vi "模式插入面板.vi"(10 "面板地址":string(combo), 11 "模式选择":string(combo)) -> ()   [LabVIEW 2019]
panel:
  in  "模式input":T1 {"pannel"."ID" format="%02x"}
  in  "节点列表":T2(array[cluster])
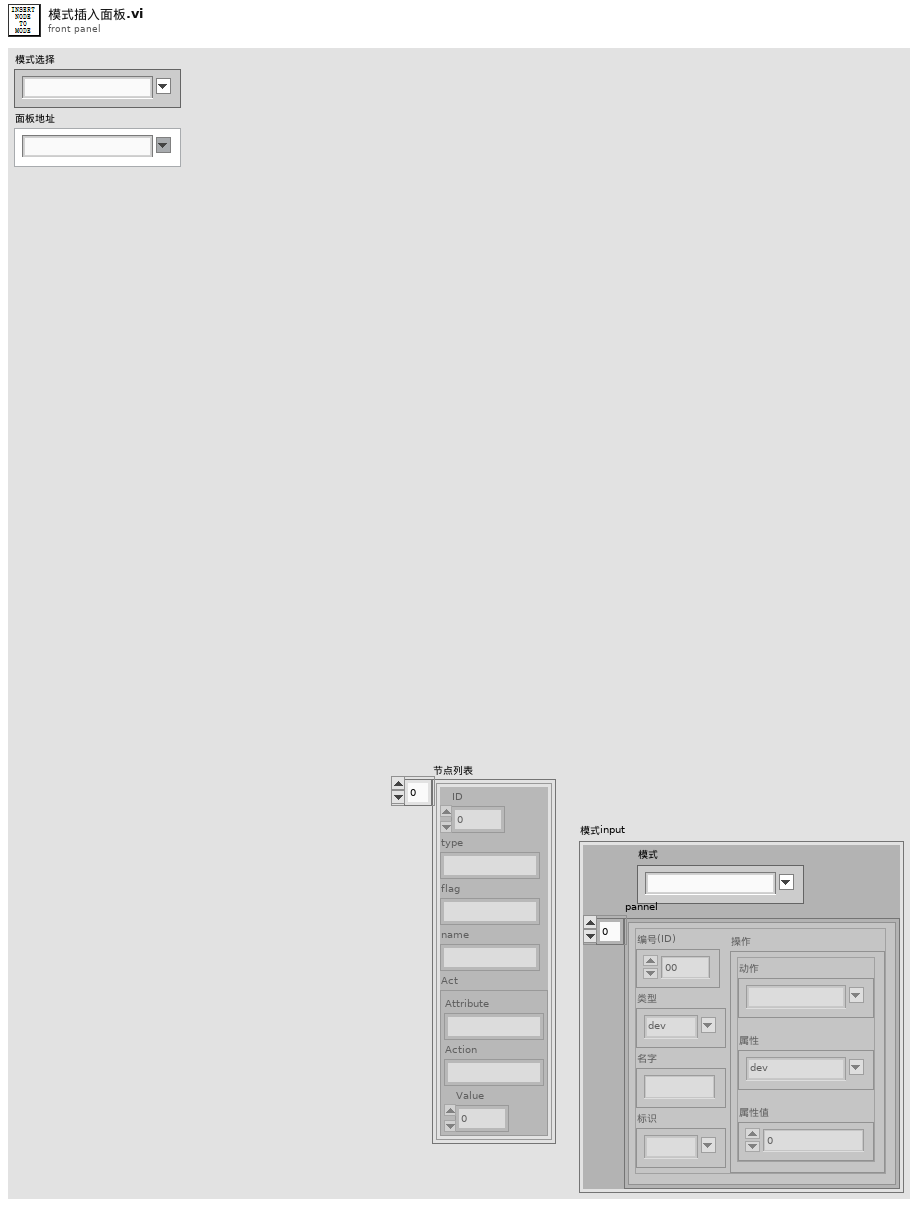
[diagram p1: front panel]
types:
  T1 = cluster{"模式":string, "pannel":cluster{"ID":u8, "type":string, "flag":string, "name":string, "Act":cluster{"Attribute":string, "Action":string, "Value":dbl}}[]}
  T2 = cluster{"ID":u8, "type":string, "flag":string, "name":string, "Act":cluster{"Attribute":string, "Action":string, "Value":dbl}}[]
  T3 = cluster{"模式":string, "数组":cluster{"地址":string, "名字":string, "编号":string, "动作":string, "拼接":string}[]}
  T4 = cluster{"地址":string, "名字":string, "编号":string, "动作":string, "拼接":string}[]
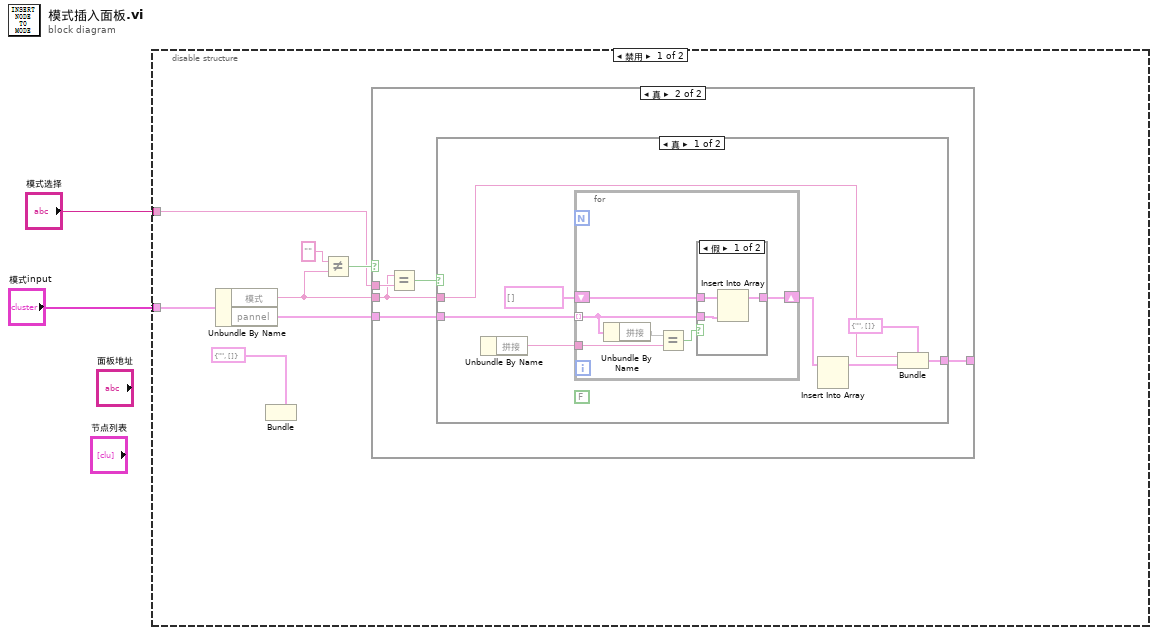
[diagram p0: block diagram]
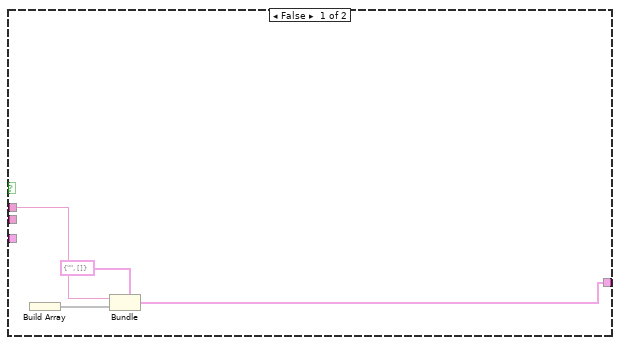
[diagram p2: hidden frame]
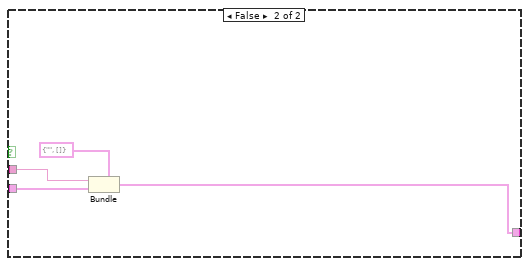
[diagram p4: hidden frame]
diagram:
  n1 = disable-structure shown="禁用" {
    disable-tunnel: "模式input" -> [w5 _]
    disable-tunnel: "模式选择" -> [w3 _]
    frame Disabled {
      n2 = Unbundle By Name(w5) -> ("模式"=w8:string, "pannel"=w9:T2)
      n3 = Bundle(cluster=T1 {"模式"="", "pannel"=[]} ("模式input")) -> ()  [unwired: 2 in, 1 out]
      n4 = Not Equal?(x="", y=w8) -> (x != y?=w6:bool)
      n5 = case shown="真" w6 {
        tunnel: w3 -> [w10 w18]
        tunnel: w9 -> [_ w16]
        tunnel: w8 -> [_ w15]
        tunnel: [w11 w14] -> _
        frame False {
          n6 = Build Array() -> (w12:void[])  [unwired: 1 in]
          n7 = Bundle(cluster=T3 {"模式"="", "数组"=[]} ("模式"), "模式"=w10, "数组"=w12) -> (w11:T3)
        }
        frame True {
          n8 = Equal?(x=w15, y=w18) -> (x = y?=w17:bool)
          n9 = case shown="真" w17 {
            tunnel: w16 -> [w26 w38]
            tunnel: w15 -> [w23 w39]
            tunnel: [w22 w37] -> w14
            frame True {
              (unwired) FALSE
              n10 = Unbundle By Name() -> ("拼接"=w19:string)  [unwired: 1 in]
              n11 = for {
                tunnel: w26 -> [w28] mode=indexing
                shift-right: [w29] -> w21
                shift-left: T4 [] -> [w30]
                tunnel: w19 -> [w27]
                n12 = Unbundle By Name(w28) -> ("拼接"=w32)
                n13 = Equal?(x=w32, y=w27) -> (x = y?=w31:bool)
                n14 = case shown="假" w31 {
                  tunnel: w30 -> [w34 w36]
                  tunnel: [w35 w36] -> w29
                  tunnel: w28 -> [w33 _]
                  frame False {
                    n15 = Insert Into Array(array=w34, new element=w33) -> (w35:T4)  [unwired: 1 in]
                  }
                  frame True {
                  }
                }
              }
              n16 = Insert Into Array(array=w21) -> (w20:T4)  [unwired: 2 in]
              n17 = Bundle(cluster=T3 {"模式"="", "数组"=[]} ("模式"), "模式"=w23, "数组"=w20) -> (w22:T3)
            }
            frame False {
              n18 = Bundle(cluster=T3 {"模式"="", "数组"=[]} ("模式"), "模式"=w39, "数组"=w38) -> (w37:T3)
            }
          }
        }
      }
    }
    frame Enabled {
    }
  }
